vi "target_setup.vi"(0 "Flattened Parameters in":string[](array[string]), 1 "error in (no error)":errorcluster) -> (2 "Pass":bool, 3 "Flattened Parameters out":string[](array[string]), 4 "error out":errorcluster)   [LabVIEW 2010]
uses:
  CommonSubVIs/Framework/Flattened_Array/Test Parameter Enum.ctl
  <vilib>/nisyscfg/Initialize (String).vi
  <vilib>/nisyscfg/Find Hardware.vi
  <vilib>/nisyscfg/Close (System).vi
  <vilib>/nisyscfg/Save Changes (Hardware).vi
  <vilib>/nisyscfg/Close (Hardware).vi
  <vilib>/nisyscfg/nisyscfg.lvlib
  Program Files (x86)/National Instruments/LabVIEW 2010/resource/objmgr/nisysapi.rc
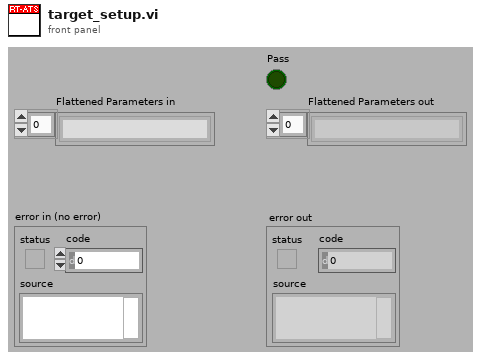
[diagram p1: front panel]
types:
  T1 = typedef "Test Parameter Enum.ctl" = enum16{"Main Test Target IP", "Main Test Target Name", "Main Test Target Alias", "Main Host IP", "Default Target Alias", "Default Target Host Name", "Dafault Target IP Address", "Dafault Target LV Date", "Available Targets", "Target Alias by Index", "Target IP by Alias", "Target IP by  Index", "Current Iteration", "Total Iterations", "Test Project Name", "Current Test Result", "Current Test Name", "Current Test Logical Path", "Test Folder", "Configuration Name", "Configuration Index", "Total Configurations", "Performance Values", "Result Paragraphs", "Connector Pane", "Avoid?", "Avoid Reason", "Case Name", "Case #", "Total Cases", "Case Data", "Disable reason"}
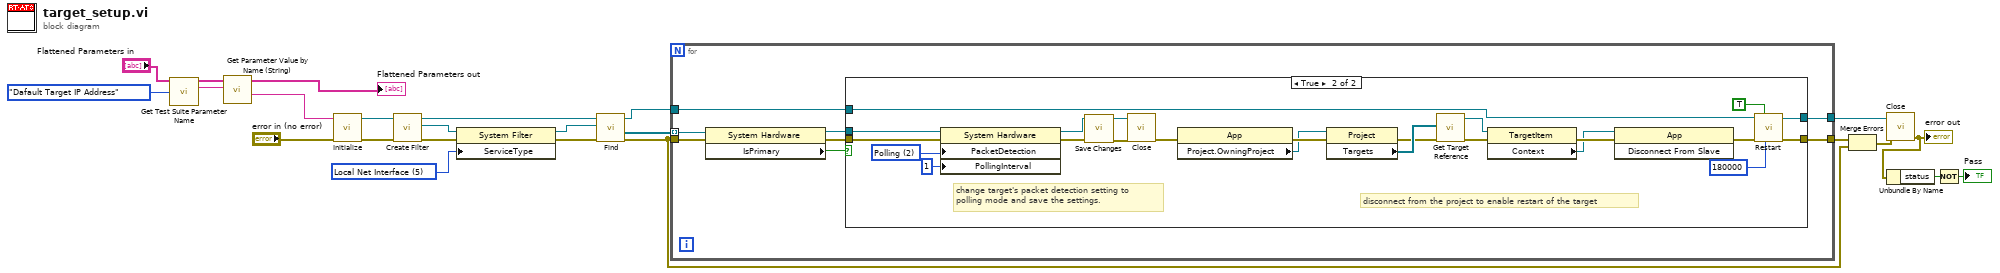
[diagram p0: block diagram]
diagram:
  w21 = u32 5 items=["NI Network Resource", "NI Real-Time", "NI System Configuration", "NI Web Interface", "Local System", "Local Net Interface", "Local Time Keeper", "Local Time Reference", "LXI Instrument"] ("Service Type")
  n1 = call "Get Test Suite Parameter Name.vi"("Test Suite Parameter"=Test_Parameter_Enum."Dafault Target IP Address") -> ("Parameter Name"=w12:string)  [unwired: 13 in, 1 out]
  n2 = call "Get Parameter Value by Name (String).vi"("Parameter"=w12, "Parameter Array in"="Flattened Parameters in") -> ("Value"=w4:string, "Parameter Array Out"=→"Flattened Parameters out":string[])  [unwired: 6 in, 1 out]
  n3 = call-poly <vilib>:"Initialize.vi"("error in (no error)"="error in (no error)", "target (localhost)"=w4) -> ("error out"=w1:errorcluster, "session out"=w3:refnum<k21>)  [unwired: 7 in, 1 out]
  n4 = call <vilib>:"Create Filter.vi"("error in (no error)"=w1, "session in"=w3) -> ("error out"=w22:errorcluster, "filter out"=w23:refnum<k20>, "session out"=w19:refnum<k21>)  [unwired: 7 in]
  n5 = property class="System Filter"(reference=w23, error in=w22, "ServiceType"=w21) -> (reference out=w20:refnum<k20>, error out=w18:errorcluster)
  n6 = call-poly <vilib>:"Find.vi"("error in (no error)"=w18, "filter in"=w20, "session in"=w19) -> ("error out"=w8:errorcluster, "resources out"=w16:refnum<k20>[], "session out"=w17:refnum<k21>)  [unwired: 5 in, 1 out]
  n7 = for {
    tunnel: w8 -> [w31]
    tunnel: w17 -> [w27]
    tunnel: w16 -> [w26] mode=indexing
    tunnel: [w25] -> w15
    tunnel: [w24] -> w14
    n8 = property class="System Hardware"(reference=w26, error in=w31) -> (reference out=w28:refnum<k20>, error out=w29:errorcluster, "IsPrimary"=w30:bool)
    n9 = case shown="True" w30 {
      tunnel: w29 -> [w33 w56]
      tunnel: w28 -> [_ w55]
      tunnel: w27 -> [w32 w52]
      tunnel: [w33 w53] -> w24
      tunnel: [w32 w46] -> w25
      frame False {
      }
      frame True {
        w54 = u32 2 items=["Interrupt"=1, "Polling"=2] ("Network Adapters:TCP/IP:Packet Detection")
        # "change target's packet detection setting to \npolling mode and save the settings."
        # "disconnect from the project to enable restart of the target"
        n10 = property class="System Hardware"(reference=w55, error in=w56, "PacketDetection"=w54, "PollingInterval"=u32 1 ("Network Adapters:TCP/IP:Polling Interval")) -> (reference out=w48:refnum<k20>, error out=w49:errorcluster)
        n11 = call-poly <vilib>:"Save Changes.vi"("error in (no error)"=w49, "resource in"=w48) -> ("error out"=w50:errorcluster, "resource out"=w47:refnum<k20>)  [unwired: 6 in, 2 out]
        n12 = call-poly <vilib>:"Close.vi"("error in (no error)"=w50, "resource in"=w47) -> ("error out"=w35:errorcluster)  [unwired: 9 in]
        n13 = property class="App"(error in=w35) -> (error out=w44:errorcluster, "Project.OwningProject"=w43:refnum<vi>)  [unwired: 1 in, 1 out]
        n14 = property class="Project"(reference=w43, error in=w44) -> (error out=w41:errorcluster, "Targets"=w42:refnum<vi>[])  [unwired: 1 out]
        n15 = call "Get Target Reference.vi"("error in"=w41, "Targets"=w42) -> ("error out"=w39:errorcluster, "RT Target Refnum"=w40:refnum<vi>)  [unwired: 1 in, 5 out]
        n16 = property class="TargetItem"(reference=w40, error in=w39) -> (error out=w38:errorcluster, "Context"=w37:refnum<vi>)  [unwired: 1 out]
        n17 = invoke class="App" method="Disconnect From Slave"(reference=w37, error in=w38) -> (error out=w36:errorcluster)  [unwired: 1 in, 2 out]
        n18 = call <vilib>:"Restart.vi"("timeout msec (90000)"=u32 180000, "wait until complete (T)"=TRUE, "error in (no error)"=w36, "session in"=w52) -> ("error out"=w53:errorcluster, "session out"=w46:refnum<k21>)  [unwired: 5 in, 1 out]
      }
    }
  }
  n19 = Merge Errors(w14, w8) -> (w9:errorcluster)
  n20 = call-poly <vilib>:"Close.vi"("error in (no error)"=w9, "session in"=w15) -> ("error out"=w7:errorcluster)  [unwired: 9 in]
  "error out" <- w7
  n21 = Unbundle By Name(w7) -> ("status"=w6:bool)
  n22 = Not(x=w6) -> (.not. x?=→"Pass":bool)
